vi "PutArray.vi"(8 "error in (no error)":errorcluster, 10 "Array":variant, 11 "MsgPackSerializer in":refnum<class "MsgPackSerializer.lvclass">) -> (0 "error out":errorcluster, 3 "MsgPackSerializer out":refnum<class "MsgPackSerializer.lvclass">)   [LabVIEW 2015, in "MsgPackSerializer.lvclass"]
uses:
  MsgPackSerializer.lvclass
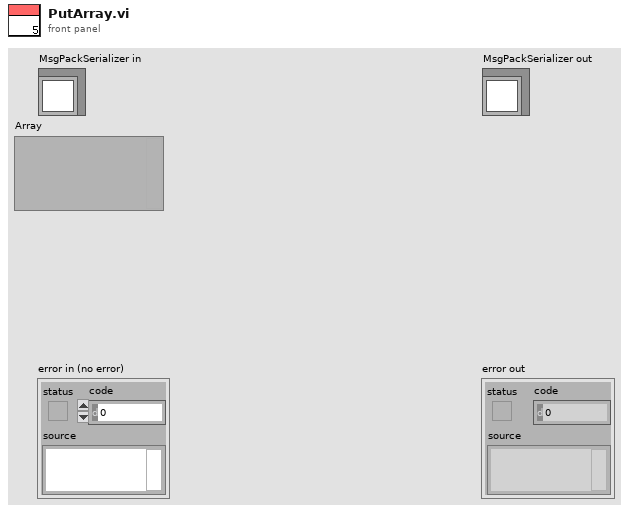
[diagram p1: front panel]
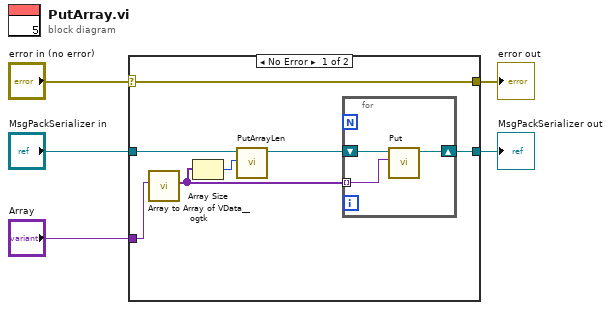
[diagram p0: block diagram]
diagram:
  n1 = case shown="No Error" "error in (no error)" {
    selector: "error in (no error)" -> [w12 w17]
    tunnel: [w12 w17] -> w4
    tunnel: [w9 w16] -> w2
    tunnel: "MsgPackSerializer in" -> [w8 w16]
    tunnel: "Array" -> [w11 _]
    frame No Error {
      n2 = call <userlib>:"Array to Array of VData__ogtk.vi"("MultiD Array"=w11) -> ("1D Array of Variants"=w10:variant[])  [unwired: 9 in, 1 out]
      n3 = Array Size(array=w10) -> (size(s)=w6:i32)
      n4 = call "PutArrayLen.vi"("len"=w6, "MsgPackSerializer in"=w8) -> ("MsgPackSerializer out"=w7:refnum<class "MsgPackSerializer.lvclass">)  [unwired: 8 in, 1 out]
      n5 = for {
        tunnel: w10 -> [w15] mode=indexing
        shift-right: [w13] -> w9
        shift-left: w7 -> [w14]
        n6 = call "Put.vi"("Data"=w15, "MsgPackSerializer in"=w14) -> ("MsgPackSerializer out"=w13:refnum<class "MsgPackSerializer.lvclass">)  [unwired: 8 in, 1 out]
      }
    }
    frame Error {
    }
  }
  "error out" <- w4
  "MsgPackSerializer out" <- w2
